vi "Encoder Input.vi"() -> ()   [LabVIEW 2009]
uses:
  <vilib>/DAQmx/read.llb/DAQmx Read (Digital U8 1Chan 1Samp).vi
panel:
  out "ft3 per Hour":dbl
  out "ft3":dbl
  in  "ft3 Per Rotation":dbl format="%_3g"
  in  "Ticks Per Rotation":dbl=400.0
  out "dT":dbl
  out "Threes":i16
  out "Twos":i16
  out "Ones":i16
  out "Time, Encoder, Tick":dbl[][](array[numeric])
  in  "Number of Samples":i32=100
  in  "Data Sample Period(10s)":u32=10
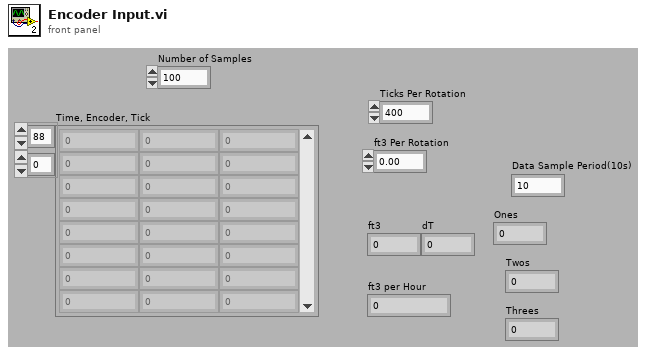
[diagram p1: front panel]
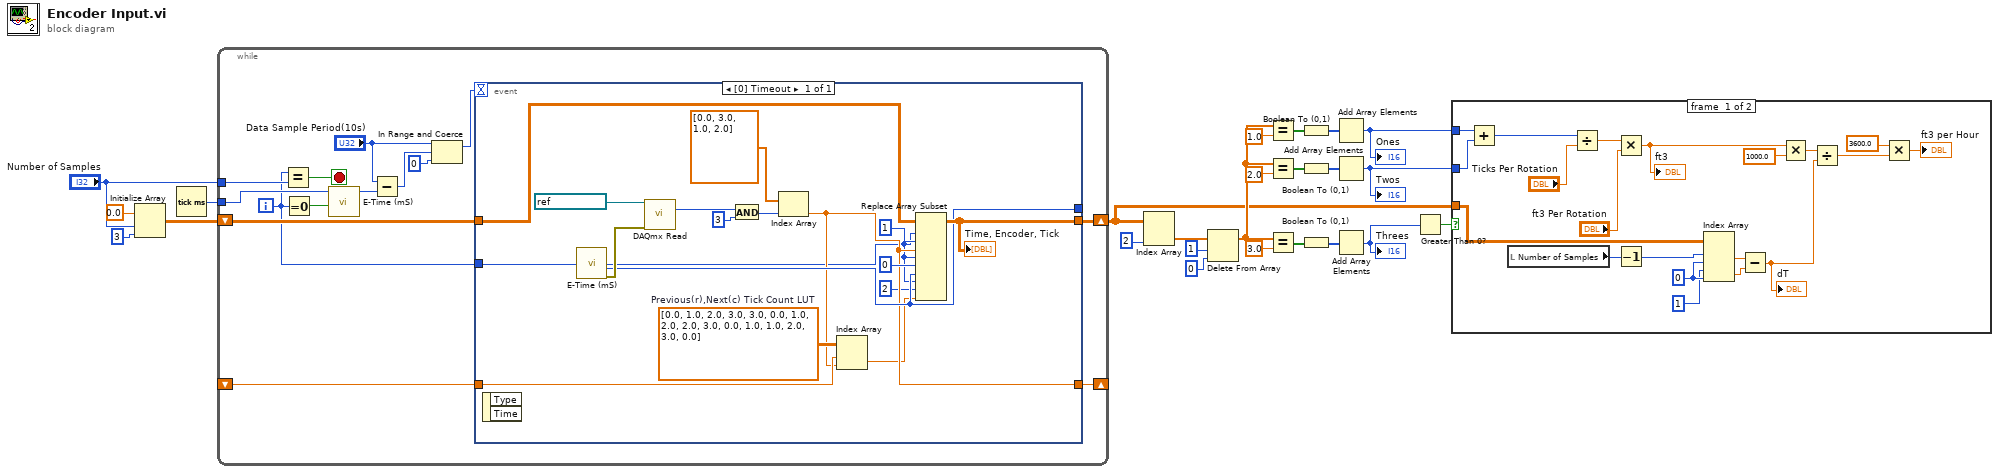
[diagram p0: block diagram]
diagram:
  n1 = Initialize Array(0.0 ("element"), "Number of Samples", 3 ("dimension size")) -> (w21:dbl[][])
  n2 = Tick Count (ms)() -> (millisecond timer value=w20:u32)
  n3 = while {
    tunnel: "Number of Samples" -> [w37]
    shift-right: [w35] -> w1
    shift-left: w21 -> [w36]
    tunnel: w20 -> [w29]
    shift-right: [w26] -> _
    shift-left: _ -> [w25]
    i -> [w27]
    stop <- w38 stop-if-true
    n4 = Equal?(x=w27, y=w37) -> (x = y?=w38:bool)
    n5 = Equal To 0?(x=w27) -> (x = 0?=w28:bool)
    n6 = call "E-Time (mS).vi"("Enter Start Time(mS)"=w29, "Reset"=w28) -> ("Time Since Last Run(mS)"=w32:u32)  [unwired: 7 in, 2 out]
    n7 = Subtract(x="Data Sample Period(10s)", y=w32) -> (x-y=w34:u32)
    n8 = In Range and Coerce(upper limit="Data Sample Period(10s)", x=w34, lower limit=u32 0) -> (coerced(x)=w30:u32)  [unwired: 1 out]
    n9 = event shown="[0] Timeout" {
      selector: _ -> [_]
      dyn-events: _ -> [_]
      timeout: w30 -> [_]
      tunnel: [w44] -> _
      tunnel: w36 -> [w52]
      tunnel: w27 -> [w39]
      tunnel: [w47] -> w35
      tunnel: [w42] -> w26
      tunnel: w25 -> [w43]
      event [0] Timeout {
        w45 = dbl[][] [[0.0, 1.0, 2.0, 3.0], [3.0, 0.0, 1.0, 2.0], [2.0, 3.0, 0.0, 1.0], [1.0, 2.0, 3.0, 0.0]]  # Previous(r),Next(c) Tick Count LUT
        n10 = event-data() -> ()  [unwired: 1 in, 2 out]
        n11 = call "E-Time (mS).vi"() -> ("error out"=w46:errorcluster, "Elapsed Time (mS)"=w44:u32)  [unwired: 9 in, 1 out]
        n12 = call-poly <vilib>:"DAQmx Read.vi"("task/channels in"=refnum<k21> "PortRead", "error in"=w46) -> ("data"=w54:u8)  [unwired: 11 in, 2 out]
        n13 = And(x=w54, y=u8 3) -> (x .and. y?=w51:u8)
        n14 = Index Array(array=dbl[] [0.0, 3.0, 1.0, 2.0], index=w51) -> (element=w42:dbl)
        n15 = Index Array(array=w45, index (row)=w43, index (col)=w42) -> (element=w41:dbl)
        n16 = Replace Array Subset(array=w52, new element #1=w42, index (row) #1=w39, index (col) #1=1 ("disabled index (col)"), new element #2=w44, index (row) #2=w39, index (col) #2=0 ("disabled index (col)"), new element #3=w41, index (row) #3=w39, index (col) #3=2 ("index (row)")) -> (w47:dbl[][])
        "Time, Encoder, Tick" <- w47
      }
    }
  }
  n17 = Index Array(array=w1, index (col)=2 ("disabled index (col)")) -> (element=w2:dbl[])  [unwired: 1 in]
  n18 = Delete From Array(array=w2, length=1, index=0) -> (array with subset deleted=w9:dbl[])  [unwired: 1 out]
  n19 = Equal?(x=w9, y=1.0) -> (x = y?=w17:bool[])
  n20 = Equal?(x=w9, y=2.0) -> (x = y?=w10:bool[])
  n21 = Equal?(x=w9, y=3.0) -> (x = y?=w12:bool[])
  n22 = Boolean To (0,1)(Boolean=w17) -> (0, 1=w16:i16[])
  n23 = Boolean To (0,1)(Boolean=w10) -> (0, 1=w15:i16[])
  n24 = Boolean To (0,1)(Boolean=w12) -> (0, 1=w11:i16[])
  n25 = Add Array Elements(numeric array=w16) -> (sum=w3:i16)
  "Ones" <- w3
  n26 = Add Array Elements(numeric array=w15) -> (sum=w4:i16)
  "Twos" <- w4
  n27 = Add Array Elements(numeric array=w11) -> (sum=w5:i16)
  "Threes" <- w5
  n28 = Greater Than 0?(x=w5) -> (x > 0?=w6:bool)
  n29 = case shown="False" w6 {
    tunnel: w4 -> [w75 _]
    tunnel: w3 -> [w74 _]
    tunnel: w1 -> [w73 _]
    frame #0 {
      w63 = 0 ("disabled index (row)")
      n30 = Add(x=w74, y=w75) -> (x+y=w69:i16)
      n31 = local read "Number of Samples"() -> (w57:i32)
      n32 = Divide(x=w69, y="Ticks Per Rotation") -> (x/y=w67:dbl)
      n33 = Multiply(x=w67, y="ft3 Per Rotation") -> (x*y=w61:dbl)
      "ft3" <- w61
      n34 = Decrement(x=w57) -> (x-1=w56:i32)
      n35 = Index Array(array=w73, index (row) #1=w56, index (col) #1=w63, index (row) #2=1 ("disabled index (col)"), index (col) #2=w63) -> (element #1=w71:dbl, element #2=w72:dbl)
      n36 = Subtract(x=w71, y=w72) -> (x-y=w58:dbl)
      "dT" <- w58
      n37 = Multiply(x=w61, y=1000.0) -> (x*y=w59:dbl)
      n38 = Divide(x=w59, y=w58) -> (x/y=w66:dbl)
      n39 = Multiply(x=3600.0, y=w66) -> (x*y=→"ft3 per Hour":dbl)
    }
    frame #1 {
      # "Too Fast to Read Accurately"
    }
  }
